vi "Execute.vi"(8 "error in":errorcluster, 10 "Stop CMD in":refnum<class "Stop CMD.lvclass">, 11 "Instrument In":refnum<class "Instrument.lvclass">) -> (0 "error out":errorcluster, 3 "Instrument Out":refnum<class "Instrument.lvclass">)   [LabVIEW 2013, in "Stop CMD.lvclass"]
uses:
  Stop CMD.lvclass
  Instrument.lvclass
  state.ctl
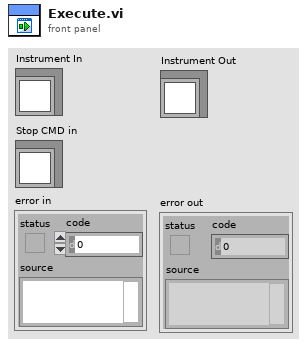
[diagram p1: front panel]
types:
  T1 = typedef "Instrument.lvclass/state.ctl" = enum8{"Configure", "Acquire", "Wait", "Quit", "Handle Error", "NOOP"}
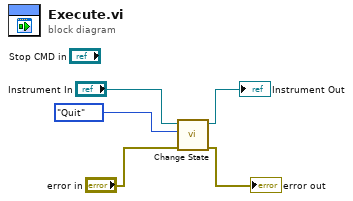
[diagram p0: block diagram]
diagram:
  n1 = call "Change State.vi"("error in"="error in", "instr state"=state."Quit", "Instrument in"="Instrument In") -> ("error out"=→"error out":errorcluster, "Instrument out"=→"Instrument Out":refnum<class "Instrument.lvclass">)  [unwired: 7 in]
